vi "XIPIN_IBERT_Virtex6_GTH_(ChipScope_Pro_-_IBERT)_2_03_a.vi"   [LabVIEW 2017]
doc: "The ChipScope(TM) Pro Integrated Bit Error Ratio Tester (IBERT) core for Virtex(R)-6 GTH is a customizable core that can be used to evaluate and monitor the health of Virtex-6 GTHTransceivers.\n------------------------------------\n<b>Need License</b> : No"
uses:
  <vilib>/rvi/XilinxIP/XIPIN_XNode/niFpgaXIPIN.xnode
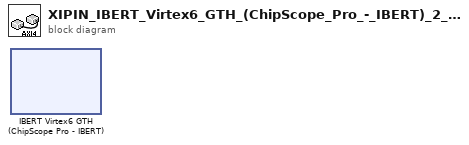
[diagram p0: block diagram]
diagram:
  n1 = xnode ("IBERT Virtex6 GTH (ChipScope Pro - IBERT)")() -> ()
